vi "oa_Polar Create Attribute.vi"(0 "channel name":string, 1 "order":dbl, 2 "x-axis units":T1 items=["Time (s)"=0, "Frequency-CB (Hz)"=1, "Frequency-CPB (Hz)"=1248, "Frequency-Arbitrary (Hz)"=2357, "Quefrency (s)"=2, "Revolutions (rev)"=3, "Order"=4, "Speed (RPM)"=11, "Speed (rad/s)"=21, "Index"=65535], 3 "rotation direction":u16, 4 "probe angle [deg]":u16, 5 "error in (no error)":errorcluster) -> (14 "attribute out":variant, 19 "error out":errorcluster)   [LabVIEW 2017]
uses:
  <vilib>/addons/_NISVFA/_Shared subVIs/Controls/svc_X-Axis Units.ctl
  <vilib>/addons/Sound and Vibration/Order Analysis/Misc/SVMS Attribute.ctl
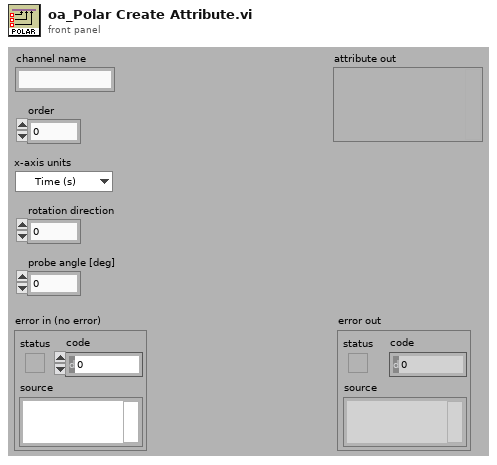
[diagram p1: front panel]
types:
  T1 = typedef "svc_X-Axis Units.ctl" = u16
  T2 = typedef "SVMS Attribute.ctl" = u16
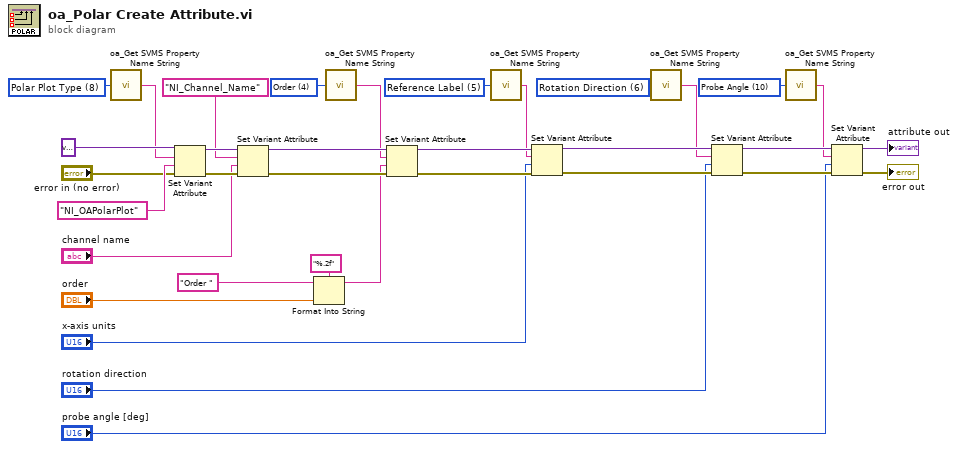
[diagram p0: block diagram]
diagram:
  w2 = T2 10 items=["Pulse / Revolution", "Slope", "Threshold", "Hysteresis", "Order", "Reference Label", "Rotation Direction", "Pair String", "Polar Plot Type", "Sample Per Revolution", "Probe Angle", "Probe Angle X", "Probe Angle Y", "X Axis Unit", "OTB Plot Type"] ("attribute")
  w4 = T2 6 items=["Pulse / Revolution", "Slope", "Threshold", "Hysteresis", "Order", "Reference Label", "Rotation Direction", "Pair String", "Polar Plot Type", "Sample Per Revolution", "Probe Angle", "Probe Angle X", "Probe Angle Y", "X Axis Unit", "OTB Plot Type"] ("attribute")
  w6 = T2 5 items=["Pulse / Revolution", "Slope", "Threshold", "Hysteresis", "Order", "Reference Label", "Rotation Direction", "Pair String", "Polar Plot Type", "Sample Per Revolution", "Probe Angle", "Probe Angle X", "Probe Angle Y", "X Axis Unit", "OTB Plot Type"] ("attribute")
  w8 = T2 4 items=["Pulse / Revolution", "Slope", "Threshold", "Hysteresis", "Order", "Reference Label", "Rotation Direction", "Pair String", "Polar Plot Type", "Sample Per Revolution", "Probe Angle", "Probe Angle X", "Probe Angle Y", "X Axis Unit", "OTB Plot Type"] ("attribute")
  w10 = T2 8 items=["Pulse / Revolution", "Slope", "Threshold", "Hysteresis", "Order", "Reference Label", "Rotation Direction", "Pair String", "Polar Plot Type", "Sample Per Revolution", "Probe Angle", "Probe Angle X", "Probe Angle Y", "X Axis Unit", "OTB Plot Type"] ("attribute")
  n1 = call <vilib>:"oa_Get SVMS Property Name String.vi"("attribute"=w10) -> ("attribute name"=w9:string)  [unwired: 4 in]
  n2 = Set Variant Attribute(Variant=variant ("attribute"), name=w9, value="NI_OAPolarPlot" ("name"), error in="error in (no error)") -> (Variant out=w27:variant, error out=w28:errorcluster)  [unwired: 1 out]
  n3 = Set Variant Attribute(Variant=w27, name="NI_Channel_Name", value="channel name", error in=w28) -> (Variant out=w24:variant, error out=w25:errorcluster)  [unwired: 1 out]
  n4 = Format Into String(format string="%.2f", initial string="Order " ("string"), "order") -> (resulting string=w11:string)  [unwired: 1 in, 1 out]
  n5 = call <vilib>:"oa_Get SVMS Property Name String.vi"("attribute"=w8) -> ("attribute name"=w7:string)  [unwired: 4 in]
  n6 = Set Variant Attribute(Variant=w24, name=w7, value=w11, error in=w25) -> (Variant out=w22:variant, error out=w23:errorcluster)  [unwired: 1 out]
  n7 = call <vilib>:"oa_Get SVMS Property Name String.vi"("attribute"=w6) -> ("attribute name"=w5:string)  [unwired: 4 in]
  n8 = Set Variant Attribute(Variant=w22, name=w5, value="x-axis units", error in=w23) -> (Variant out=w31:variant, error out=w32:errorcluster)  [unwired: 1 out]
  n9 = call <vilib>:"oa_Get SVMS Property Name String.vi"("attribute"=w4) -> ("attribute name"=w3:string)  [unwired: 4 in]
  n10 = Set Variant Attribute(Variant=w31, name=w3, value="rotation direction", error in=w32) -> (Variant out=w29:variant, error out=w30:errorcluster)  [unwired: 1 out]
  n11 = call <vilib>:"oa_Get SVMS Property Name String.vi"("attribute"=w2) -> ("attribute name"=w1:string)  [unwired: 4 in]
  n12 = Set Variant Attribute(Variant=w29, name=w1, value="probe angle [deg]", error in=w30) -> (Variant out=→"attribute out":variant, error out=→"error out":errorcluster)  [unwired: 1 out]
